vi "MinusMean2D (SubVI).vi"(8 "Image Pixels":dbl[][](array[numeric])) -> (1 "standard deviation":dbl format="%0.2f", 2 "mean":dbl format="%0.2f", 4 "Array":dbl[][](array[numeric]))   [LabVIEW 2011, in "OfflineTracker.lvlib"]
uses:
  OfflineTracker.lvlib
  <vilib>/Analysis/NI_AALBase.lvlib
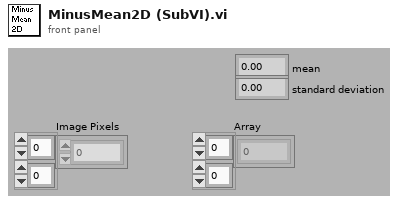
[diagram p1: front panel]
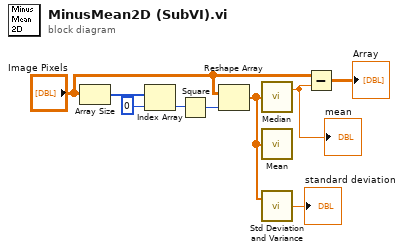
[diagram p0: block diagram]
diagram:
  n1 = Array Size(array="Image Pixels") -> (size(s)=w6:i32[])
  n2 = Index Array(array=w6, index=0) -> (element=w7:i32)
  n3 = Square(x=w7) -> (x^2=w8:i32)
  n4 = Reshape Array("Image Pixels", w8) -> (w2:dbl[])
  n5 = call <vilib>:"Median.vi"("X"=w2) -> ("median"=w1:dbl)  [unwired: 1 out]
  "mean" <- w1
  n6 = call <vilib>:"Mean.vi"("X"=w2) -> ()  [unwired: 2 out]
  n7 = call <vilib>:"Std Deviation and Variance.vi"("X"=w2) -> ("standard deviation"=→"standard deviation":dbl)  [unwired: 1 in, 2 out]
  n8 = Subtract(x="Image Pixels", y=w1) -> (x-y=→"Array":dbl[][])
